vi "niFpgaHandshakeEmulation.vi"(0 "name":string, 2 "Node Link":cluster{"VIRef":refnum<vi>, "UID":i32}, 5 "fourWireIn":bool, 7 "data in":variant, 9 "Method":T1, 11 "Directly In SCTL":bool, 12 "Local? (F)":bool, 13 "Ref In wired (F)":bool) -> (6 "fourWireOut":bool, 8 "data out":variant)   [LabVIEW 2017]
uses:
  <vilib>/rvi/DataTransferAndStorage/Container/Common/niFpgaContainerMethod.ctl
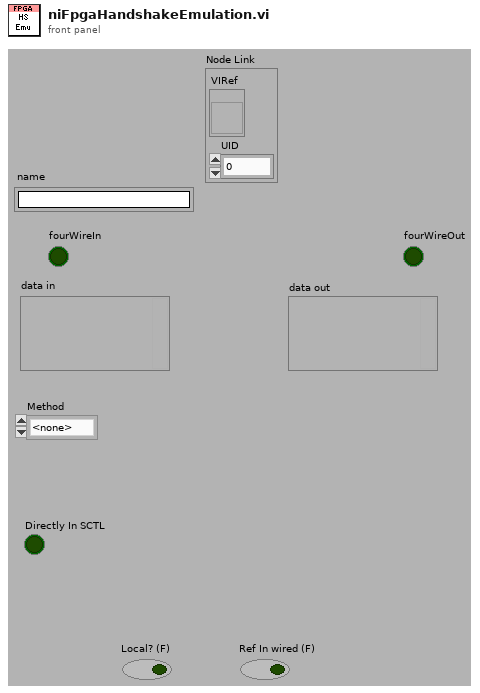
[diagram p1: front panel]
types:
  T1 = typedef "niFpgaContainerMethod.ctl" = enum16{"<none>", "write", "read", "clear", "getNumberOfElementsToWrite", "getNumberOfElementsToRead", "enable", "disable", "flushAndDisable", "getStreamState", "readA", "readB", "dramWrite", "dramWriteWithByteEnables", "dramRequestData", "dramRetrieveData", "readWithoutAcknowledge", "acknowledge", "writeUsingHandshaking", "readUsingHandshaking", "flush"}
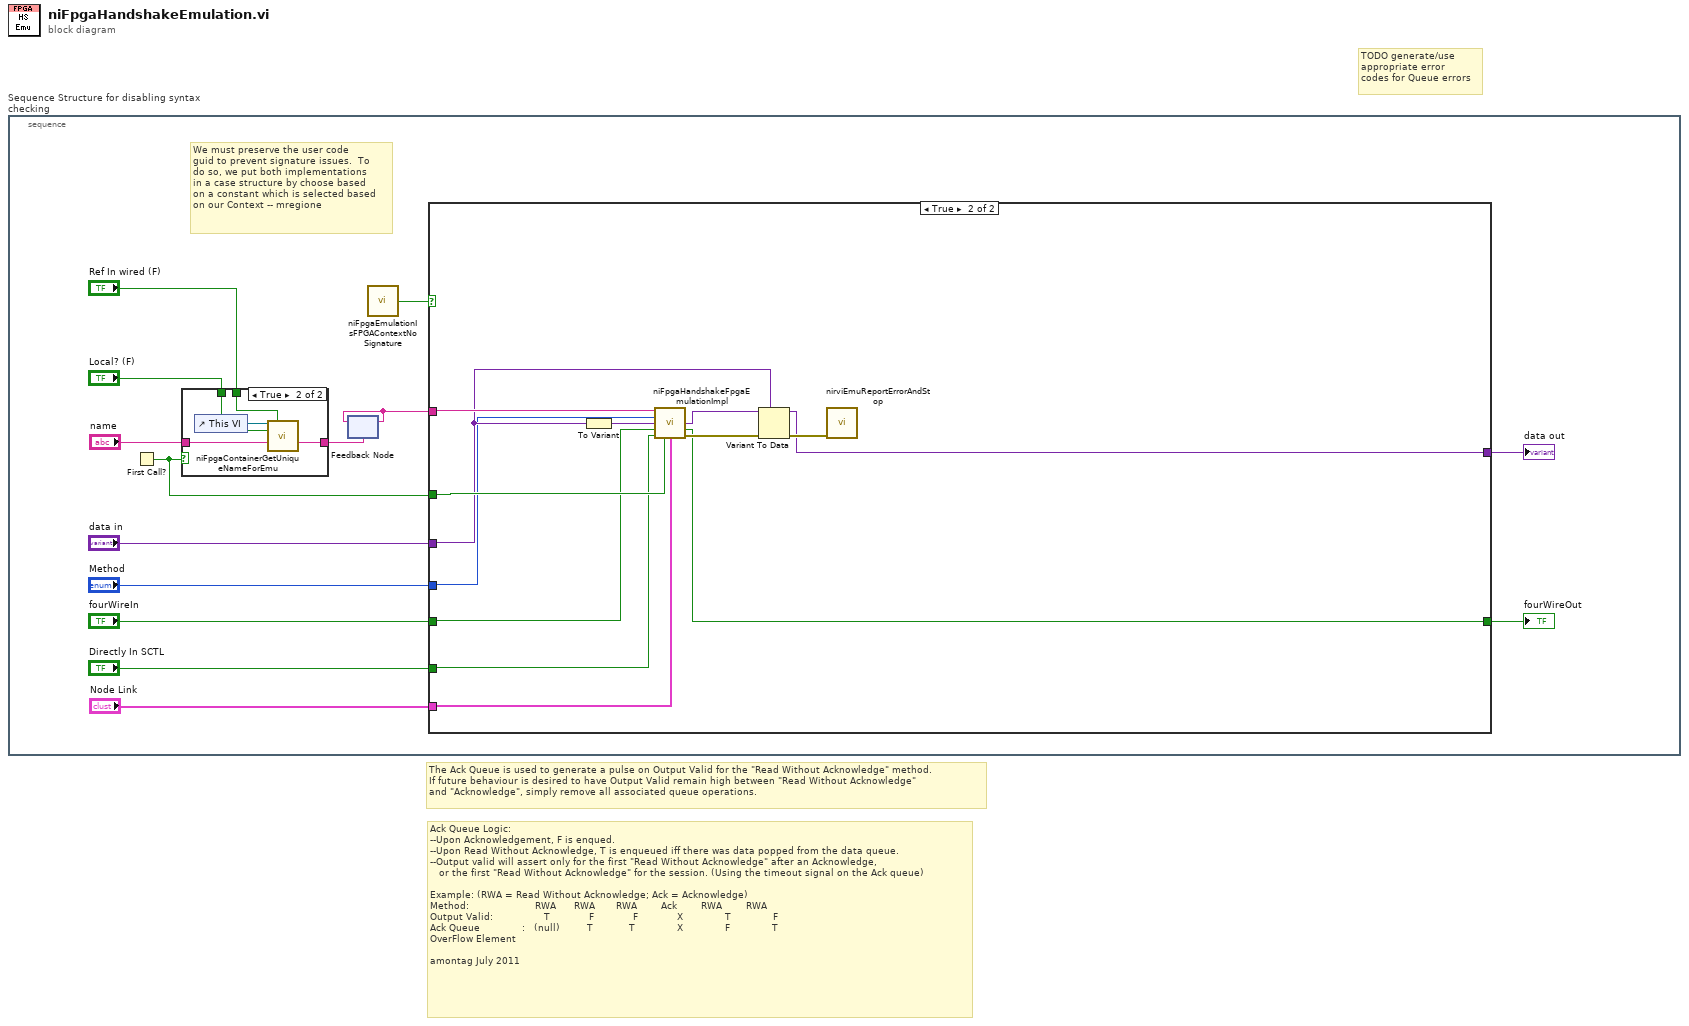
[diagram p0: block diagram]
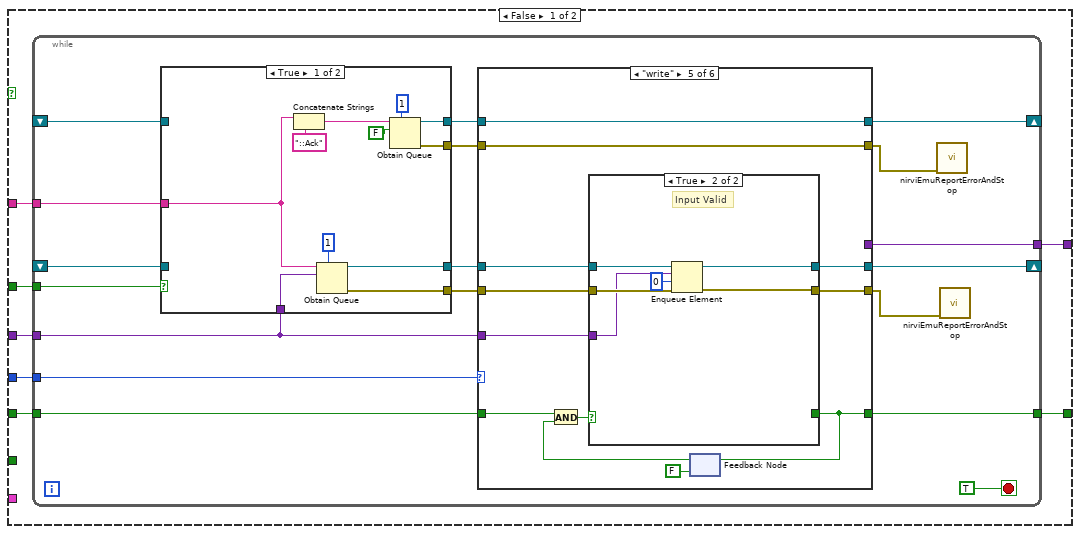
[diagram p2: hidden frame]
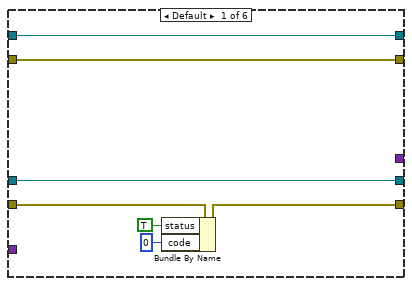
[diagram p3: hidden frame]
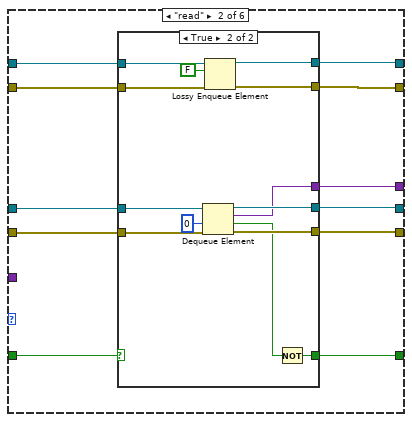
[diagram p4: hidden frame]
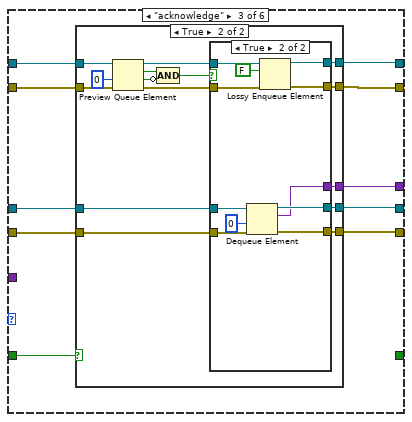
[diagram p6: hidden frame]
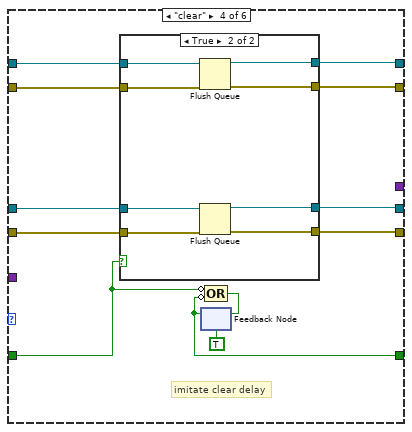
[diagram p9: hidden frame]
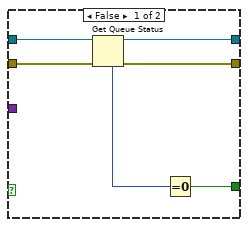
[diagram p11: hidden frame]
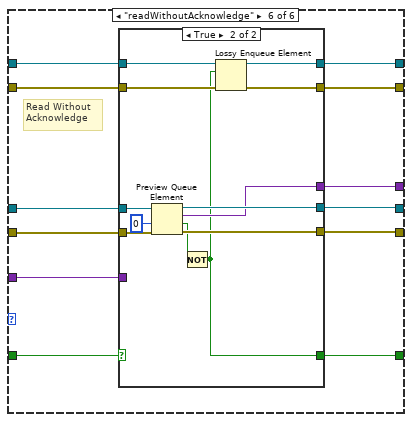
[diagram p12: hidden frame]
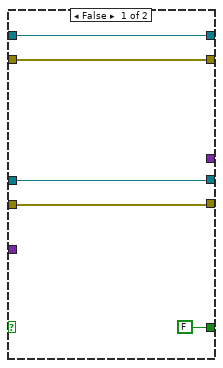
[diagram p13: hidden frame]
diagram:
  # "TODO generate/use \nappropriate error\ncodes for Queue errors"
  # "Ack Queue Logic:\n--Upon Acknowledgement, F is enqued.\n--Upon Read Without Acknowledge, T is enqueued iff there was data popped from the data queue.\n--Output valid will assert only for the first \"Read Without Acknowledge\" after an Acknowledge, \n   or the first \"Read Without Acknowledge\" for the session. (Using the timeout signal on the Ack queue)\n\nExample: (RWA = Read Without Acknowledge; Ack = Acknowledge)\nMethod:                      RWA      RWA       RWA        Ack        RWA        RWA\nOutput Valid:                 T             F             F             X              T              F\nAck Queue              :   (null)         T            T              X              F              T         \nOverFlow Element\n\namontag July 2011"
  # "The Ack Queue is used to generate a pulse on Output Valid for the \"Read Without Acknowledge\" method.\nIf future behaviour is desired to have Output Valid remain high between \"Read Without Acknowledge\" \nand \"Acknowledge\", simply remove all associated queue operations."
  n1 = stacked-sequence "Sequence Structure for disabling syntax checking" {
    frame #0 {
      # "We must preserve the user code\nguid to prevent signature issues.  To\ndo so, we put both implementations\nin a case structure by choose based\non a constant which is selected based\non our Context -- mregione"
      n2 = First Call?() -> (First Call?: T/F=w4:bool)
      n3 = case shown="True" w4 {
        tunnel: "name" -> [_ w225]
        tunnel: "Ref In wired (F)" -> [_ w224]
        tunnel: "Local? (F)" -> [_ w223]
        tunnel: [_ w222] -> w6
        frame False {
        }
        frame True {
          n4 = control-ref of="This VI"() -> (w226:refnum<vi>)
          n5 = call <vilib>:"niFpgaContainerGetUniqueNameForEmu.vi"("parent VI"=w226, "ref in wired"=w224, "local"=w223, "name in"=w225) -> ("name out"=w222:string)  [unwired: 11 in]
        }
      }
      n6 = feedback #1(w6) -> (w5:string)
      n7 = feedback-in #1(w5) -> ()
      n8 = call <vilib>:"niFpgaEmulationIsFPGAContextNoSignature.vi"() -> ("Is Fpga Context?"=w1:bool)  [unwired: 15 in]
      n9 = case shown="True" w1 {
        tunnel: "data in" -> [w21 w215]
        tunnel: "Method" -> [w20 w214]
        tunnel: "fourWireIn" -> [w19 w213]
        tunnel: [w18 w210] -> w11
        tunnel: [w17 w209] -> w10
        tunnel: w5 -> [w16 w217]
        tunnel: w4 -> [w15 w216]
        tunnel: "Node Link" -> [_ w211]
        tunnel: "Directly In SCTL" -> [_ w212]
        frame False {
          n10 = while {
            shift-right: [w37] -> _
            shift-left: _ -> [w38]
            shift-right: [w36] -> _
            shift-left: _ -> [w35]
            tunnel: w21 -> [w28]
            tunnel: w20 -> [w27]
            tunnel: w19 -> [w26]
            tunnel: w16 -> [w25]
            tunnel: [w24] -> w18
            tunnel: [w23] -> w17
            tunnel: w15 -> [w22]
            stop <- TRUE stop-if-true
            n11 = case shown="True" w22 {
              tunnel: w25 -> [w196 _]
              tunnel: [w198 _] -> w33
              tunnel: w28 -> [w205 _]
              tunnel: [w204 w208] -> w34
              tunnel: w38 -> [_ w208]
              tunnel: [w199 w207] -> w32
              tunnel: w35 -> [_ w207]
              tunnel: [w197 _] -> w31
              frame True {
                n12 = Concatenate Strings(w196, "::Ack" ("string")) -> (w200:string)
                n13 = Obtain Queue(max queue size (-1, unlimited)=1, name (unnamed)=w196, element data type=w205) -> (queue out=w204:refnum<queue>, error out=w198:errorcluster)  [unwired: 2 in, 1 out]
                n14 = Obtain Queue(max queue size (-1, unlimited)=1, name (unnamed)=w200, element data type=FALSE) -> (queue out=w199:refnum<queue>, error out=w197:errorcluster)  [unwired: 2 in, 1 out]
              }
              frame False {
              }
            }
            n15 = case shown="\"write\"" w27 {
              tunnel: w34 -> [w46 w53 w81 w128 w152 w174]
              tunnel: w33 -> [w43 w55 w83 w130 w154 w176]
              tunnel: [w46 w52 w80 w127 w151 w173] -> w37
              tunnel: [w42 w54 w82 w129 w153 w175] -> w30
              tunnel: w26 -> [_ w57 w84 w121 w144 w178]
              tunnel: [_ w56 _ w120 w147 w177] -> w24
              tunnel: [_ w51 w79 _ _ w171] -> w23
              tunnel: w28 -> [_ _ _ _ w150 w172]
              tunnel: w32 -> [w45 w50 w78 w124 w149 w170]
              tunnel: [w45 w47 w75 w122 w149 w169] -> w36
              tunnel: [w44 w49 w77 w123 w148 w167] -> w29
              tunnel: w31 -> [w44 w48 w76 w125 w148 w168]
              frame Default {
                n16 = Bundle By Name(cluster=w43, "status"=TRUE, "code"=0) -> (w42:errorcluster)
              }
              frame "read" {
                n17 = case shown="True" w57 {
                  tunnel: [_ w70] -> w56
                  tunnel: w55 -> [w60 w66]
                  tunnel: [w60 w74] -> w54
                  tunnel: w53 -> [w61 w72]
                  tunnel: [w61 w71] -> w52
                  tunnel: [_ w68] -> w51
                  tunnel: w50 -> [w58 w67]
                  tunnel: [w59 w65] -> w49
                  tunnel: w48 -> [w59 w63]
                  tunnel: [w58 w64] -> w47
                  frame False {
                  }
                  frame True {
                    n18 = Dequeue Element(queue=w72, timeout in ms (-1)=0, error in (no error)=w66) -> (queue out=w71:refnum<queue>, element=w68:variant, timed out?=w69:bool, error out=w74:errorcluster)
                    n19 = Lossy Enqueue Element(queue=w67, element=FALSE, error in (no error)=w63) -> (queue out=w64:refnum<queue>, error out=w65:errorcluster)  [unwired: 2 out]
                    n20 = Not(x=w69) -> (.not. x?=w70:bool)
                  }
                }
              }
              frame "acknowledge" {
                n21 = case shown="True" w84 {
                  tunnel: w83 -> [w87 w99]
                  tunnel: [w87 w103] -> w82
                  tunnel: w81 -> [w88 w102]
                  tunnel: [w88 w101] -> w80
                  tunnel: [_ w100] -> w79
                  tunnel: w78 -> [w85 w93]
                  tunnel: [w86 w98] -> w77
                  tunnel: w76 -> [w86 w96]
                  tunnel: [w85 w97] -> w75
                  frame False {
                  }
                  frame True {
                    n22 = Preview Queue Element(queue=w93, timeout in ms (-1)=0, error in (no error)=w96) -> (queue out=w92:refnum<queue>, element=w90:bool, timed out?=w89:bool, error out=w95:errorcluster)
                    n23 = Compound Arithmetic op=AND(w90, invert w89) -> (w91:bool)
                    n24 = case shown="True" w91 {
                      tunnel: [w104 w118] -> w103
                      tunnel: w102 -> [w105 w116]
                      tunnel: [w105 w115] -> w101
                      tunnel: [_ w114] -> w100
                      tunnel: w99 -> [w104 w113]
                      tunnel: [w106 w112] -> w98
                      tunnel: [w107 w111] -> w97
                      tunnel: w95 -> [w106 w109]
                      tunnel: w92 -> [w107 w108]
                      frame False {
                      }
                      frame True {
                        n25 = Dequeue Element(queue=w116, timeout in ms (-1)=0, error in (no error)=w113) -> (queue out=w115:refnum<queue>, element=w114:variant, error out=w118:errorcluster)  [unwired: 1 out]
                        n26 = Lossy Enqueue Element(queue=w108, element=FALSE, error in (no error)=w109) -> (queue out=w111:refnum<queue>, error out=w112:errorcluster)  [unwired: 2 out]
                      }
                    }
                  }
                }
              }
              frame "clear" {
                # "imitate clear delay"
                n27 = case shown="True" w121 {
                  tunnel: w130 -> [w133 w139]
                  tunnel: [w133 w140] -> w129
                  tunnel: w128 -> [w134 w142]
                  tunnel: [w134 w141] -> w127
                  tunnel: w125 -> [w131 w138]
                  tunnel: w124 -> [w132 w136]
                  tunnel: [w131 w137] -> w123
                  tunnel: [w132 w135] -> w122
                  frame False {
                  }
                  frame True {
                    n28 = Flush Queue(queue=w136, error in (no error)=w138) -> (queue out=w135:refnum<queue>, error out=w137:errorcluster)  [unwired: 1 out]
                    n29 = Flush Queue(queue=w142, error in (no error)=w139) -> (queue out=w141:refnum<queue>, error out=w140:errorcluster)  [unwired: 1 out]
                  }
                }
                n30 = feedback #2(TRUE ("fourWireIn")) -> (w120:bool)
                n31 = Compound Arithmetic op=OR(invert w121, invert w120) -> (w119:bool)
                n32 = feedback-in #2(w119) -> ()
              }
              frame "write" {
                n33 = feedback #3(FALSE) -> (w145:bool)
                n34 = And(x=w144, y=w145) -> (x .and. y?=w146:bool)
                n35 = case shown="True" w146 {
                  tunnel: [w156 _] -> w147
                  tunnel: w154 -> [w158 w166]
                  tunnel: [w157 w161] -> w153
                  tunnel: w152 -> [w160 w164]
                  tunnel: [w159 w163] -> w151
                  tunnel: w150 -> [_ w162]
                  frame False {
                    n36 = Get Queue Status(queue=w160, error in (no error)=w158) -> (queue out=w159:refnum<queue>, error out=w157:errorcluster, # elements in queue=w155:i32)  [unwired: 1 in, 5 out]
                    n37 = Equal To 0?(x=w155) -> (x = 0?=w156:bool)
                  }
                  frame True {
                    # "Input Valid"
                    n38 = Enqueue Element(queue=w164, element=w162, timeout in ms (-1)=0, error in (no error)=w166) -> (queue out=w163:refnum<queue>, error out=w161:errorcluster)  [unwired: 1 out]
                  }
                }
                n39 = feedback-in #3(w147) -> ()
              }
              frame "readWithoutAcknowledge" {
                # "Read Without \nAcknowledge"
                n40 = case shown="True" w178 {
                  tunnel: [FALSE ("shakeOut") w184] -> w177
                  tunnel: w176 -> [w182 w187]
                  tunnel: [w182 w193] -> w175
                  tunnel: w174 -> [w181 w195]
                  tunnel: [w181 w194] -> w173
                  tunnel: w172 -> [_ _]
                  tunnel: [_ w191] -> w171
                  tunnel: w170 -> [w180 w190]
                  tunnel: [w180 w189] -> w169
                  tunnel: w168 -> [w179 w186]
                  tunnel: [w179 w188] -> w167
                  frame False {
                  }
                  frame True {
                    n41 = Preview Queue Element(queue=w195, timeout in ms (-1)=0, error in (no error)=w187) -> (queue out=w194:refnum<queue>, element=w191:variant, timed out?=w185:bool, error out=w193:errorcluster)
                    n42 = Not(x=w185) -> (.not. x?=w184:bool)
                    n43 = Lossy Enqueue Element(queue=w190, element=w184, error in (no error)=w186) -> (queue out=w189:refnum<queue>, error out=w188:errorcluster)  [unwired: 2 out]
                  }
                }
              }
            }
            n44 = call <vilib>:"nirviEmuReportErrorAndStop.vi"("error to report"=w29) -> ()  [unwired: 3 in, 12 out]
            n45 = call <vilib>:"nirviEmuReportErrorAndStop.vi"("error to report"=w30) -> ()  [unwired: 3 in, 12 out]
          }
        }
        frame True {
          n46 = To Variant(anything=w215) -> (Variant=w219:variant)
          n47 = call <vilib>:"niFpgaHandshakeFpgaEmulationImpl.vi"("Name"=w217, "Method"=w214, "Data In"=w219, "Four-wire In"=w213, "Directly In SCTL"=w212, "First Call"=w216, "Node Link"=w211) -> ("Data Out"=w220:variant, "Four-wire Out"=w210:bool, "Error Out"=w221:errorcluster)  [unwired: 6 in]
          n48 = Variant To Data(error in=w221, type=w215, Variant=w220) -> (data=w209:variant, error out=w218:errorcluster)
          n49 = call <vilib>:"nirviEmuReportErrorAndStop.vi"("error to report"=w218) -> ()  [unwired: 1 in, 14 out]
        }
      }
      "fourWireOut" <- w11
      "data out" <- w10
    }
  }
